vi "ZLIB Open Write File__ogtk.vi"(5 "local extra data":string, 6 "password (none)":string, 7 "raw mode (F)":bool, 8 "error in (no error)":errorcluster, 9 "file info":T1={"version"=0, "version needed"=0, "encrypted"=FALSE, "flag"=4294967295, "compression"=0, "dos date"=0, "crc"=0, "compressed size"=0, "uncompressed size"=0, "extra info"="", "file comment"="", "disk num start"=0, "internal fa"=0, "external fa"=0, "file timestamp"=0} {"file timestamp" format="%<%H:%M:%S\n%d/%m/%Y>T"; "external fa" format="%.0x"; "internal fa" format="%.0x"; "crc" format="%.0x"}, 10 "filename":string, 11 "zip Refnum":T2) -> (0 "error out":errorcluster, 3 "zip Refnum out":T2)   [LabVIEW 2019]
doc: "Creates a new entry in the ZIP archive for a new file."
uses:
  ZLIB Compress File Info__ogtk.ctl
  <userlib>/_OpenG.lib/lvzip/lvzlib.dll
  ZLIB Zip Handle__ogtk.ctl
  ZLIB File Info__ogtk.ctl
panel:
  # "Please visit http://www.OpenG.org to learn about the\nOpen Source LabVIEW software movement.\n\nNOTICE -- YOU MUST LEAVE THIS NOTICE IN PLACE.  PER THE TERMS OF THE LICENSE BELOW, YOU MAY SUBLICENSE THIS SOFTWARE \nIN ANY WAY THAT DOES NOT CONFLICT WITH THIS LICENSE.\n\n### BSD License (http://www.opensource.org/licenses/bsd-license.php) Begin ###\n \nCopyright (C) 2002-2004 Rolf Kalbermatter rolf.kalbermatter@citeng.com\nCopyright (C) 2002 Jim Kring jim@jimkring.com\n\nAll rights reserved.\n\nRedistribution and use in source and binary forms, with or without modification, are permitted provided that the following conditions are met:\n\n    * Redistributions of source code must retain the above copyright notice, this list of conditions and the following disclaimer.\n    * Redistributions in binary form must reproduce the above copyright notice, this list of conditions and the following disclaimer in the \n       documentation and/or other materials provided with the distribution.\n    * Neither the name of SciWare, James Kring, Inc., nor the names of its contributors may be used to endorse or promote products derived \n       from this software without specific prior written permission.\n\nTHIS SOFTWARE IS PROVIDED BY THE COPYRIGHT HOLDERS AND CONTRIBUTORS \"AS IS\" AND ANY EXPRESS OR IMPLIED WARRANTIES, \nINCLUDING, BUT NOT LIMITED TO, THE IMPLIED WARRANTIES OF MERCHANTABILITY AND FITNESS FOR A PARTICULAR PURPOSE ARE \nDISCLAIMED. IN NO EVENT SHALL THE COPYRIGHT OWNER OR CONTRIBUTORS BE LIABLE FOR ANY DIRECT, INDIRECT, INCIDENTAL,\n SPECIAL, EXEMPLARY, OR CONSEQUENTIAL DAMAGES (INCLUDING, BUT NOT LIMITED TO, PROCUREMENT OF SUBSTITUTE GOODS OR \nSERVICES; LOSS OF USE, DATA, OR PROFITS; OR BUSINESS INTERRUPTION) HOWEVER CAUSED AND ON ANY THEORY OF LIABILITY, \nWHETHER IN CONTRACT, STRICT LIABILITY, OR TORT (INCLUDING NEGLIGENCE OR OTHERWISE) ARISING IN ANY WAY OUT OF THE USE \nOF THIS SOFTWARE, EVEN IF ADVISED OF THE POSSIBILITY OF SUCH DAMAGE.\n\n### BSD License End ###"
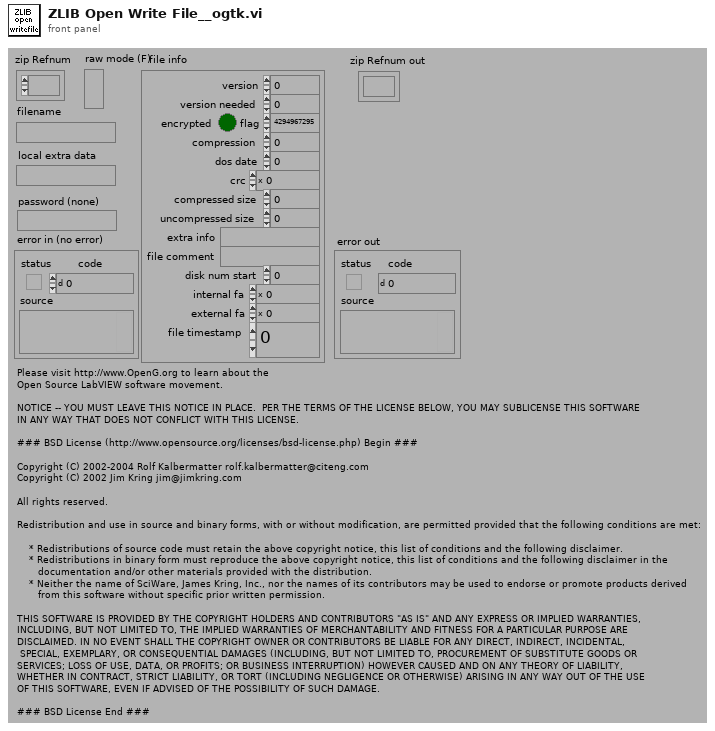
[diagram p1: front panel]
types:
  T1 = typedef "ZLIB File Info__ogtk.ctl" = cluster{"version":u32, "version needed":u32, "encrypted":bool, "flag":u32, "compression":i32, "dos date":u32, "crc":u32, "compressed size":u32, "uncompressed size":u32, "extra info":string, "file comment":string, "disk num start":u32, "internal fa":u32, "external fa":u32, "file timestamp":u32}
  T2 = typedef "ZLIB Zip Handle__ogtk.ctl" = refnum<k1>
  T3 = typedef "ZLIB Compress File Info__ogtk.ctl" = cluster{"date time":cluster{"sec":i32, "min":i32, "hour":i32, "mday":i32, "mon":i32, "year":i32}, "dosTime":u32, "internal fa":u32, "external fa":u32}
  T4 = cluster{"second":i32, "minute":i32, "hour":i32, "day of month":i32, "month":i32, "year":i32, "day of week":i32, "day of year":i32, "is DST":i32}
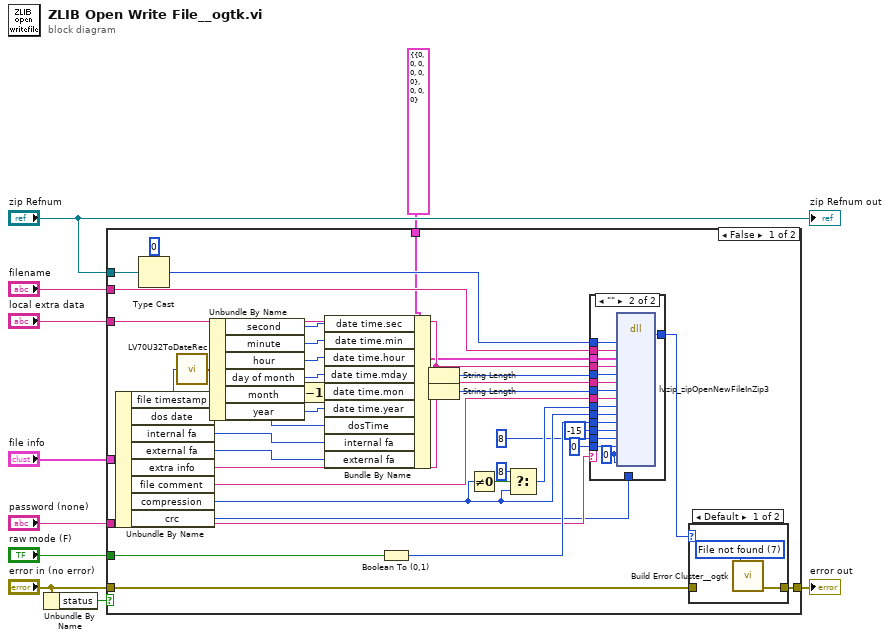
[diagram p0: block diagram]
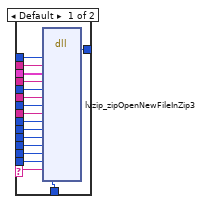
[diagram p2: hidden frame]
diagram:
  n1 = Unbundle By Name("error in (no error)") -> ("status"=w9:bool)
  n2 = case shown="False" w9 {
    tunnel: "error in (no error)" -> [w47 w85]
    tunnel: [w46 w85] -> w10
    tunnel: "zip Refnum" -> [w43 _]
    tunnel: "filename" -> [w42 _]
    tunnel: "file info" -> [w41 _]
    tunnel: "local extra data" -> [w37 _]
    tunnel: T3 {"date time"={"sec"=0, "min"=0, "hour"=0, "mday"=0, "mon"=0, "year"=0}, "dosTime"=0, "internal fa"=0, "external fa"=0} ("file info") -> [w30 _]
    tunnel: "password (none)" -> [w12 _]
    tunnel: "raw mode (F)" -> [w17 _]
    frame False {
      n3 = Unbundle By Name(w41) -> ("file timestamp"=w34:u32, "dos date"=w32:u32, "internal fa"=w31:u32, "external fa"=w33:u32, "extra info"=w21:string, "file comment"=w19:string, "compression"=w18:i32, "crc"=w11:u32)
      n4 = Type Cast(type=u32 0 ("unzFile"), x=w43) -> (*(type *) &x=w44:u32)
      n5 = call <vilib>:"LV70U32ToDateRec.vi"("Time"=w34) -> ("date time rec"=w22:T4)
      n6 = Unbundle By Name(w22) -> ("second"=w27:i32, "minute"=w26:i32, "hour"=w25:i32, "day of month"=w28:i32, "month"=w24:i32, "year"=w23:i32)
      n7 = Decrement(x=w24) -> (x-1=w29:i32)
      n8 = Bundle By Name(cluster=w30, "date time.sec"=w27, "date time.min"=w26, "date time.hour"=w25, "date time.mday"=w28, "date time.mon"=w29, "date time.year"=w23, "dosTime"=w32, "internal fa"=w31, "external fa"=w33) -> (w20:T3)
      n9 = Boolean To (0,1)(Boolean=w17) -> (0, 1=w16:i16)
      n10 = String Length(string=w37) -> (length=w36:i32)
      n11 = String Length(string=w21) -> (length=w35:i32)
      n12 = Not Equal To 0?(x=w18) -> (x != 0?=w40:bool)
      n13 = Select(t=8, s=w40, f=w18) -> (s? t:f=w39:i32)
      n14 = case shown="\"\"" w12 {
        selector: w12 -> [w50 _]
        tunnel: [w65 w81] -> w48
        tunnel: w44 -> [w64 w80]
        tunnel: w42 -> [w63 w79]
        tunnel: w39 -> [w56 w78]
        tunnel: w37 -> [w61 w77]
        tunnel: w36 -> [w60 w76]
        tunnel: w35 -> [w58 w75]
        tunnel: w21 -> [w59 w74]
        tunnel: w20 -> [w62 w73]
        tunnel: w19 -> [w57 w72]
        tunnel: w18 -> [w55 w71]
        tunnel: w16 -> [w54 w70]
        tunnel: -15 ("windowBits") -> [w53 w69]
        tunnel: 8 ("memLevel") -> [w52 w68]
        tunnel: 0 ("strategy") -> [w51 w67]
        tunnel: w11 -> [w49 _]
        frame Default {
          n15 = dll-call lib="C:/Program Files (x86)/National Instruments/LabVIEW 2020/user.lib/_OpenG.lib/lvzip/lvzlib.*" fn="lvzip_zipOpenNewFileInZip3"("unzFile"=w64, "fileName"=w63, "file info"=w62, "extraFieldLocal"=w61, "extraFieldLocalLen"=w60, "extraFieldGlobal"=w59, "extraFieldGlobalLen"=w58, "comment"=w57, "method"=w56, "level"=w55, "raw"=w54, "windowBits"=w53, "memLevel"=w52, "strategy"=w51, "password"=w50, "crc"=w49) -> (w65:i32)  [unwired: 19 in, 2 out]
        }
        frame "" {
          w66 = u32 0 ("password")
          n16 = dll-call lib="C:/Program Files (x86)/National Instruments/LabVIEW 2020/user.lib/_OpenG.lib/lvzip/lvzlib.*" fn="lvzip_zipOpenNewFileInZip3"("unzFile"=w80, "fileName"=w79, "file info"=w73, "extraFieldLocal"=w77, "extraFieldLocalLen"=w76, "extraFieldGlobal"=w74, "extraFieldGlobalLen"=w75, "comment"=w72, "method"=w78, "level"=w71, "raw"=w70, "windowBits"=w69, "memLevel"=w68, "strategy"=w67, "password"=w66, "crc"=w66) -> (w81:i32)  [unwired: 19 in, 2 out]
        }
      }
      n17 = case shown="Default" w48 {
        tunnel: w47 -> [_ w84]
        tunnel: [w83 w84] -> w46
        frame Default {
          w82 = 7 items=["No error", "Argument error", "Memory is full", "Out of zone", "End of file", "File already open", "Generic file I/O error", "File not found", "File permission error", "Disk is full", "Duplicate path", "Too many files open", "System feature not enabled", "Resource file not found", "Cannot add resource", "Resource not found", "Image not found", "Image memory error", "Pen does not exist", "Config type invalid", "Config token not found", "Config parse error", "Config memory error", "Bad external code format", "Bad external code offset", "External code not present", "Null window", "Destroy window error", "Null menu", "Print aborted", "Bad print record", "Print driver error", "Windows error during printing", "Memory error during printing", "Print dialog error", "Generic print error", "Invalid device refnum", "Device not found", "Device parameter error", "Device unit error", "Cannot open device", "Device call aborted", "Generic error", "Cancelled by user", "Object ID too low", "Object ID too high", "Object not in heap", "Unknown heap", "Unknown object (invalid DefProc)", "Unknown object (DefProc not in table)", "Message out of range", "Invalid (null) method", "Unknown message", "Manager call not supported", "Bad address", "Network operation in progress", "Network operation timed out", "Connection is busy", "Network attribute not supported", "Network error", "Address in use", "System out of memory", "Connection aborted", "Connection refused", "Not connected", "Already connected", "Connection closed", "Initialization error (interapplication manager)", "Bad occurrence", "Wait on unbound occurrence handler", "Occurrence queue overflow", "Datalog type conflict", "Unused", "Unrecognized type (interapplication manager)", "Memory corrupt", "Failed to make temporary DLL", "Old CIN version", "Drag socket not found", "Failed to load drop-object", "Failed to register OLE object", "Failed to release OLE object", "Format specifier type mismatch", "Unknown format specifier", "Too few format specifiers", "Too many format specifiers", "Scan failed", "Newer CIN version", "Error converting to variant", "Runtime menu error", "Password tampered", "Variant attribute not found", "Incompatible variant data type", "Event data is not available", "Event Store is not present", "Occurrence is not found", "Event Queue is not created", "Event info is not available", "Refnum passed is NULL", "Error retrieving Class GUID", "Error retrieving CoClass GUID", "Error retrieving TypeLib GUID.", "Bad built application magic bytes.", "Specific driver is different from the specific driver associated with the Logical Name.", "There is no session opened to the class driver.", "Max Error", "MAX - Error with config objects", "MAX - Error loading configuration", "MAX - Group not supported"]
          n18 = call "Build Error Cluster__ogtk.vi"("code"=w82) -> ("error out"=w83:errorcluster)  [unwired: 1 in]
        }
        frame 0 {
        }
      }
    }
    frame True {
      (unwired) u32 0 ("unzFile")
    }
  }
  "error out" <- w10
  "zip Refnum out" <- "zip Refnum"
